vi "ep_SVAF Settings Configuration.vi"(0 "spectra parameters":T2, 5 "speed estimation settings":cluster{"% overlap":dbl, "algorithm":T1}, 11 "error in (no error)":errorcluster) -> (4 "initial conditions":T3 {"zoom FFT settings"."FFT settings"."window" items=["Rectangle"=0, "Hanning"=1, "Hamming"=2, "Blackman-Harris"=3, "Exact Blackman"=4, "Blackman"=5, "Flat Top"=6, "4 Term B-Harris "=7, "7 Term B-Harris"=8, "Low Sidelobe"=9, "Blackman Nuttall"=11, "Triangle"=30, "Bartlett-Hanning"=31, "Bohman"=32, "Parzen"=33, "Welch"=34, "Kaiser"=60, "Dolph-Chebyshev"=61, "Gaussian"=62]}, 15 "error out":errorcluster)   [LabVIEW 2014, in "NI_EP_Motor Monitoring.lvlib"]
uses:
  <vilib>/addons/Electrical Power/Motor Monitoring/NI_EP_Motor Monitoring.lvlib
  <vilib>/addons/Electrical Power/Motor Monitoring/subVIs/ep_Initial Conditions for Speed Estimation.ctl
  <vilib>/addons/Electrical Power/Motor Monitoring/subVIs/ep_Demodulation Algorithm.ctl
  <vilib>/addons/Electrical Power/Motor Monitoring/subVIs/ep_Zoom FFT Settings.ctl
  <vilib>/addons/Electrical Power/Motor Monitoring/subVIs/ep_Spectra Settings.ctl
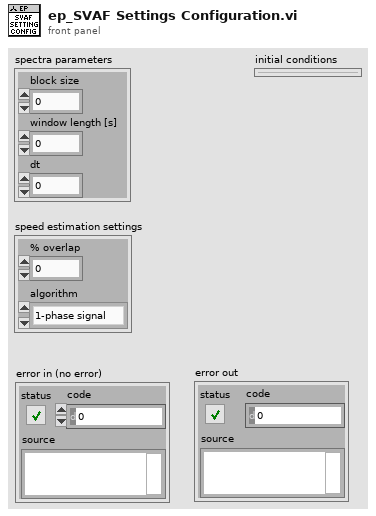
[diagram p1: front panel]
types:
  T1 = typedef "NI_EP_Motor Monitoring.lvlib/ep_Demodulation Algorithm.ctl" = enum16{"1-phase signal", "3-phase signals"}
  T2 = cluster{"block size":i32, "window length [s]":dbl, "dt":dbl}
  T3 = typedef "NI_EP_Motor Monitoring.lvlib/ep_Initial Conditions for Speed Estimation.ctl" = cluster{"SVAF state":cluster{"space vector amplitude":dbl, "hilbert state":cluster{"delay conditions":dbl[], "filter conditions":dbl[]}}, "zoom FFT state":cluster{"phase state":dbl, "zoom FFT state":cluster{"zoom settings state":cluster{"zoom":i32, "stop band attenuation":enum16{"84 dB", "96 dB", "120 dB"}, "alias protect in final transition":bool, "oversampling ratio":dbl}, "SML Decimation Filter (complex input) state":cluster{"decimation settings state":cluster{"M":i32, "stop band attenuation":enum16{"84 dB", "96 dB", "120 dB"}, "alias protect in transition band":bool, "oversampling ratio":dbl}, "counter for garbage samples state":i32, "sml_Parameter Setting for Zoom Factor state":cluster{"filter length * interpolation state":i32, "interpolation state":i32, "comb filter order state":i32, "CFIR par state":cluster{"h":dbl[], "M":i32, "N":i32}, "LFIR par state":cluster{"h":dbl[], "M":i32, "N":i32}, "CIC Stages state":i32}, "aal_CIC (complex input) state":cluster{"aal_cascaded moving average (complex input) state":cluster{"states":cdb[], "circular buffers state":cdb[][], "circular buffer counter state":i32}, "aal_moving average with decimation by order (complex input) state":cluster{"residue result state":cdb, "processed data counter state":i32}}, "sml_Cascaded Decimation Filter (complex input) CFIR state":cluster{"unprocessed data state":cdb[], "final conditions state":cdb[][], "sml_M-1 Decimator with IC (complex input) state":cluster{"coefficients in reverse order state":dbl[], "max index for coefficients state":i32}}, "sml_Cascaded Decimation Filter (complex input) LFIR state":cluster{"unprocessed data state":cdb[], "final conditions state":cdb[][], "sml_M-1 Decimator with IC (complex input) state":cluster{"coefficients in reverse order state":dbl[], "max index for coefficients state":i32}}}, "ma_SML Data Packing (complex input) state":cluster{"array getting packed state":cdb[], "last array processed state":cdb[], "index state":i32, "packing parameters state":cluster{i32, "size":i32}}}, "FFT{X} [Vrms]":cdb[]}, "speed state":cluster{"speed [RPM]":dbl, "slip":dbl}, "speed estimation settings":cluster{"% overlap":dbl, "algorithm":T1}, "filter information":cluster{"coefficients":dbl[], "order":i32}, "zoom FFT settings":T4, "last valid window":i32, "fund. frequency for averager":dbl[]}
  T4 = typedef "NI_EP_Motor Monitoring.lvlib/ep_Zoom FFT Settings.ctl" = cluster{"FFT settings":cluster{"window":u16, "Window Size":i32, "FFT Size":i32, "%overlap":dbl}, "zoom settings":cluster{"zoom":i32, "stop band attenuation":enum16{"84 dB", "96 dB", "120 dB"}, "alias protect in final transition":bool, "oversampling ratio":dbl}, "other settings":cluster{"fmod":dbl, "f0":dbl, "df":dbl, "oidx":i32, "olen":i32}, "iterations":i32, "max block size":i32, "fs":dbl}
  T5 = typedef "NI_EP_Motor Monitoring.lvlib/ep_Spectra Settings.ctl" = cluster{"number of lines":i32, "% overlap":dbl, "maximum frequency [Hz]":dbl}
  T6 = cluster{"maximum frequency [Hz]":dbl, "slip error allowance":dbl, "minimum points for peak search":dbl, "accuracy of fs":dbl, "difference?":bool, " fs harmonics order":i32, "fs forbidden range":dbl, "p3:p1 valid significance ratio":dbl, "ratio for significance weighting":dbl, "significance weighting":dbl}
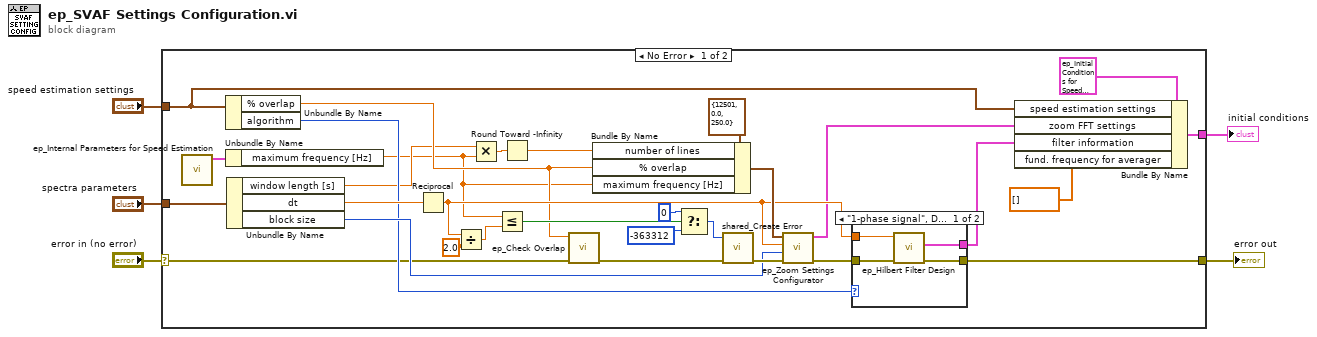
[diagram p0: block diagram]
diagram:
  n1 = case shown="No Error" "error in (no error)" {
    selector: "error in (no error)" -> [w8 w41]
    tunnel: [w35 w41] -> w4
    tunnel: "spectra parameters" -> [w20 _]
    tunnel: [w15 _] -> w1
    tunnel: "speed estimation settings" -> [w11 _]
    frame No Error {
      n2 = call <vilib>:"ep_Internal Parameters for Speed Estimation.vi"() -> ("internal parameters for speed estimation"=w10:T6)  [unwired: 11 in]
      n3 = Unbundle By Name(w11) -> ("% overlap"=w14:dbl, "algorithm"=w13:T1)
      n4 = Unbundle By Name(w10) -> ("maximum frequency [Hz]"=w9:dbl)
      n5 = Unbundle By Name(w20) -> ("window length [s]"=w12:dbl, "dt"=w19:dbl, "block size"=w18:i32)
      n6 = Reciprocal(x=w19) -> (1/x=w31:dbl)
      n7 = Divide(x=w31, y=2.0) -> (x/y=w23:dbl)
      n8 = Multiply(x=w12, y=w9) -> (x*y=w30:dbl)
      n9 = Less Or Equal?(x=w9, y=w23) -> (x <= y?=w25:bool)
      n10 = Round Toward -Infinity(1:w30) -> (0:w33:dbl)
      n11 = call <vilib>:"ep_Check Overlap.vi"("error in (no error)"=w8, "% overlap"=w14) -> ("error out"=w24:errorcluster)  [unwired: 9 in]
      n12 = Bundle By Name(cluster=T5 {"number of lines"=12501, "% overlap"=0.0, "maximum frequency [Hz]"=250.0} ("spectra settings"), "number of lines"=w33, "% overlap"=w14, "maximum frequency [Hz]"=w9) -> (w32:T5)
      n13 = Select(t=0 ("error code (0)"), s=w25, f=-363312 ("error code (0)")) -> (s? t:f=w26:i32)
      n14 = call <vilib>:"shared_Create Error.vi"("error in (no error)"=w24, "error code (0)"=w26) -> ("error out"=w21:errorcluster)  [unwired: 9 in]
      n15 = call <vilib>:"ep_Zoom Settings Configurator.vi"("error in (no error)"=w21, "block size"=w18, "fs"=w31, "spectra settings"=w32) -> ("error out"=w29:errorcluster, "zoom FFT settings"=w17:T4)  [unwired: 6 in]
      n16 = case shown="\"1-phase signal\", Default" w13 {
        tunnel: w31 -> [w39 _]
        tunnel: w29 -> [w38 w40]
        tunnel: [w37 w40] -> w35
        tunnel: [w36 _] -> w16
        frame "1-phase signal", Default {
          n17 = call <vilib>:"ep_Hilbert Filter Design.vi"("error in (no error)"=w38, "fs"=w39) -> ("error out"=w37:errorcluster, "Hilbert FIR filter"=w36:cluster{"h":dbl[], "delay":i32})  [unwired: 7 in, 1 out]
        }
        frame "3-phase signals" {
        }
      }
      n18 = Bundle By Name(cluster=T3 {"SVAF state"={"space vector amplitude"=0.0, "hilbert state"={"delay conditions"=[], "filter conditions"=[]}}, "zoom FFT state"={"phase state"=0.0, "zoom FFT state"={"zoom settings state"={"zoom"=0, "stop band attenuation"=enum."84 dB", "alias protect in final transition"=FALSE, "oversampling ratio"=0.0}, "SML Decimation Filter (complex input) state"={"decimation settings state"={"M"=0, "stop band attenuation"=enum."84 dB", "alias protect in transition band"=FALSE, "oversampling ratio"=0.0}, "counter for garbage samples state"=0, "sml_Parameter Setting for Zoom Factor state"={"filter length * interpolation state"=0, "interpolation state"=0, "comb filter order state"=0, "CFIR par state"={"h"=[], "M"=0, "N"=0}, "LFIR par state"={"h"=[], "M"=0, "N"=0}, "CIC Stages state"=0}, "aal_CIC (complex input) state"={"aal_cascaded moving average (complex input) state"={"states"=[], "circular buffers state"=[], "circular buffer counter state"=0}, "aal_moving average with decimation by order (complex input) state"={"residue result state"=0.0+0.0i, "processed data counter state"=0}}, "sml_Cascaded Decimation Filter (complex input) CFIR state"={"unprocessed data state"=[], "final conditions state"=[], "sml_M-1 Decimator with IC (complex input) state"={"coefficients in reverse order state"=[], "max index for coefficients state"=0}}, "sml_Cascaded Decimation Filter (complex input) LFIR state"={"unprocessed data state"=[], "final conditions state"=[], "sml_M-1 Decimator with IC (complex input) state"={"coefficients in reverse order state"=[], "max index for coefficients state"=0}}}, "ma_SML Data Packing (complex input) state"={"array getting packed state"=[], "last array processed state"=[], "index state"=0, "packing parameters state"={0, "size"=0}}}, "FFT{X} [Vrms]"=[]}, "speed state"={"speed [RPM]"=0.0, "slip"=0.0}, "speed estimation settings"={"% overlap"=0.0, "algorithm"=enum."1-phase signal"}, "filter information"={"coefficients"=[], "order"=0}, "zoom FFT settings"={"FFT settings"={"window"=0, "Window Size"=0, "FFT Size"=0, "%overlap"=0.0}, "zoom settings"={"zoom"=0, "stop band attenuation"=enum."84 dB", "alias protect in final transition"=FALSE, "oversampling ratio"=0.0}, "other settings"={"fmod"=0.0, "f0"=0.0, "df"=0.0, "oidx"=0, "olen"=0}, "iterations"=0, "max block size"=0, "fs"=0.0}, "last valid window"=0, "fund. frequency for averager"=[]} ("initial conditions"), "speed estimation settings"=w11, "zoom FFT settings"=w17, "filter information"=w16, "fund. frequency for averager"=dbl[] []) -> (w15:T3)
    }
    frame Error {
    }
  }
  "error out" <- w4
  "initial conditions" <- w1
